vi "Wheel Control.vi"   [LabVIEW 2015, in "Wheel.lvlib"]
uses:
  <userlib>/836-Library/Motion_Control/Shooter_Wheel/Wheel.lvlib
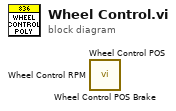
[diagram p0: block diagram]
diagram:
  n1 = call <userlib>:"Wheel Control POS Brake.vi"() -> ()  [unwired: 12 in]
  n2 = call <userlib>:"Wheel Control POS.vi"() -> ()  [unwired: 12 in]
  n3 = call <userlib>:"Wheel Control RPM.vi"() -> ()  [unwired: 12 in]
